vi "Control Type.vi"(11 "Valve in":refnum<class "DigitalControl.lvclass">) -> (2 "Valve Type":string)   [LabVIEW 2020, in "VolatusControl.lvlib" / "DigitalControl.lvclass"]
uses:
  DigitalControl.lvclass
  DigitalControl.lvclass/DigitalControl.ctl
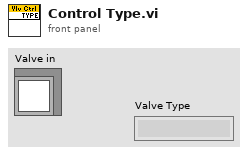
[diagram p1: front panel]
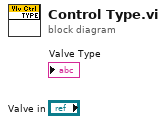
[diagram p0: block diagram]
diagram:
